vi "FRCts20_Backend_Division_DELETE.vi"(6 "Message Attributes":T4, 8 "error in (no error)":errorcluster, 10 "Data":string, 11 "Engine_Refnums":T1) -> (0 "error out":errorcluster)   [LabVIEW 2014]
doc: "Deletes a division. Called by the division/team api, and expects a division location. Does not affect any other resources, as teams and requests are not children of a division."
uses:
  FRCts20_Backend_Engine.lvlib
  FRCts20_Backend_FGVOperation.ctl
  FRCts20_Backend_API/FRCts20_Backend_API_Division.ctl
  FRCts20_Backend_API/FRCts20_Backend_API_SW.ctl
  FRCts20_Backend_API/FRCts20_Backend_API_Status.ctl
  Dependencies/Keyed Array/KeyedArray.ctl
  Dependencies/Keyed Array/Tools_KeyedArray.lvlib
  Dependencies/AMC/_SubVIs/TypeDefs/Message.ctl
  Dependencies/AMC/AMC.lvlib
  Dependencies/AMC/_SubVIs/TypeDefs/Message Queue.ctl
  <vilib>/addons/database/Connection.llb/Conn ObjectReference.ctl
  <vilib>/addons/database/NI_Database_API.lvlib
  FRCts20_Backend_EngineRefnums.ctl
  INI_Accessor/FRCts20_Backend_INI Controller.lvclass
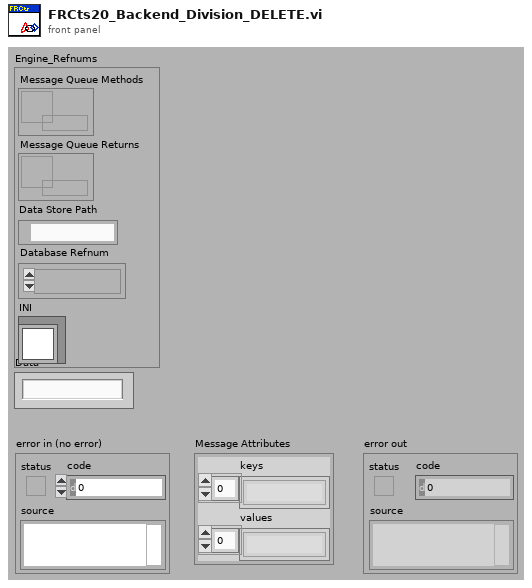
[diagram p1: front panel]
types:
  T1 = typedef "FRCts20_Backend_Engine.lvlib/FRCts20_Backend_EngineRefnums.ctl" = cluster{"Message Queue Methods":T2, "Message Queue Returns":T2, "Data Store Path":path, "Database Refnum":T3, "INI":refnum<class "FRCts20_Backend_INI Controller.lvclass">}
  T2 = typedef "AMC.lvlib/Message Queue.ctl" = refnum<queue>
  T3 = typedef "NI_Database_API.lvlib/Conn ObjectReference.ctl" = refnum<k1>
  T4 = typedef "Tools_KeyedArray.lvlib/KeyedArray.ctl" = cluster{"keys":string[], "values":string[]}
  T5 = typedef "FRCts20_Backend_API.lvlib/FRCts20_Backend_API_Division.ctl" = cluster{"Location":string, "Team":u32[], "APIReturn":string, "RootCmd":enum16{"Issues", "Software", "All"}, "SWType":T6, "Status":T7, "Competition":string}
  T6 = typedef "FRCts20_Backend_API.lvlib/FRCts20_Backend_API_SW.ctl" = string
  T7 = typedef "FRCts20_Backend_API.lvlib/FRCts20_Backend_API_Status.ctl" = enum16{"Open", "In Work", "Closed"}
  T8 = typedef "FRCts20_Backend_Engine.lvlib/FRCts20_Backend_FGVOperation.ctl" = enum16{"Initialize", "EnqueueMessage", "EnqueueDataReturn", "FlushMessage", "FlushDataReturn"}
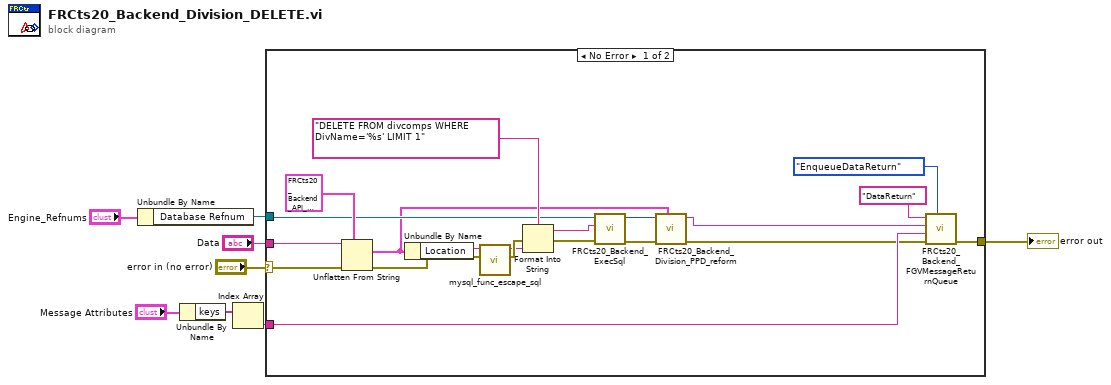
[diagram p0: block diagram]
diagram:
  n1 = Unbundle By Name("Engine_Refnums") -> ("Database Refnum"=w5:T3)
  n2 = Unbundle By Name("Message Attributes") -> ("keys"=w2:string[])
  n3 = Index Array(array=w2) -> (element=w1:string)  [unwired: 1 in]
  n4 = case shown="No Error" "error in (no error)" {
    selector: "error in (no error)" -> [w25 w29]
    tunnel: [w28 w29] -> w7
    tunnel: w5 -> [w12 _]
    tunnel: "Data" -> [w26 _]
    tunnel: w1 -> [w27 _]
    frame No Error {
      n5 = Unflatten From String(type=T5 {"Location"="", "Team"=[], "APIReturn"="", "RootCmd"=enum."Issues", "SWType"="", "Status"=enum."Open", "Competition"=""} ("Division"), binary string=w26, error in (no error)=w25) -> (value=w9:T5, error out=w24:errorcluster)  [unwired: 2 in, 1 out]
      n6 = Unbundle By Name(w9) -> ("Location"=w18:string)
      n7 = call "mysql_func_escape_sql.vi"("error in (no error)"=w24, "sqlin"=w18) -> ("error out"=w19:errorcluster, "escaped"=w17:string)  [unwired: 8 in]
      n8 = Format Into String(format string="DELETE FROM divcomps WHERE DivName='%s' LIMIT 1", error in=w19, w17) -> (resulting string=w13:string, error out=w14:errorcluster)  [unwired: 1 in]
      n9 = call "FRCts20_Backend_ExecSql.vi"("error in (no error)"=w14, "format string"=w13, "Refnum in"=w12) -> ("error out"=w15:errorcluster, "rows affected"=w16:i32)  [unwired: 6 in, 1 out]
      n10 = call "FRCts20_Backend_Division_PPD_reform.vi"("Division"=w9, "error in (no error)"=w15, "rows affected"=w16) -> ("error out"=w10:errorcluster, "data string"=w11:string)  [unwired: 7 in]
      n11 = call "FRCts20_Backend_FGVMessageReturnQueue.vi"("Operation"=FRCts20_Backend_FGVOperation."EnqueueDataReturn", "error in (no error)"=w10, "Key"=w27, "Message Value"=w11, "Message Name"="DataReturn") -> ("error out"=w28:errorcluster)  [unwired: 5 in, 1 out]
    }
    frame Error {
    }
  }
  "error out" <- w7
